vi "Orbit.vi"(11 "Input Velocities":T2) -> (3 "Output Velocities":T2)   [LabVIEW 2025]
uses:
  swerve-template/Type Definitions/Data/Robot Velocities.ctl
  <vilib>/Analysis/coordinate.llb/Angle Units.ctl
  <vilib>/Analysis/coordinate.llb/Angle Range (Degree).ctl
  <vilib>/Analysis/coordinate.llb/Wrap Angle (scalar).vi
  <vilib>/Rock Robotics/Network Tables/NT Read Integer.vi
  <vilib>/Rock Robotics/Network Tables/NT Read Float Array.vi
  <vilib>/addons/control/pid/pid.llb/PID Advanced (DBL).vi
  <vilib>/addons/control/pid/NI_PID_pid.lvlib
  <vilib>/Analysis/NI_AAL_Angle.lvlib
panel:
  in  "test values":sgl[](array[numeric])
  out "radial_vel":dbl format="%.2f"
  in  "Radius PID gains":T1={"proportional gain (Kc)"=0.01, "integral time (Ti, min)"=0.0, "derivative time (Td, min)"=0.0}
  out "radius_error":dbl
  out "desired_radius":dbl
  in  "k_radius":dbl=0.1
  out "driver_tangential_vel":dbl
  out "driver_radial_vel":dbl
  out "bearing_wrapped":dbl
  out "bearing_correction":dbl format="%.2f"
  in  "Heading PID gains":T1={"proportional gain (Kc)"=0.03, "integral time (Ti, min)"=0.0, "derivative time (Td, min)"=0.0}
  out "angular_vel_orbit":dbl
  out "desired_tangential_vel":dbl
  out "desired_radial_vel":dbl
  out "yaw":sgl
  out "curr_radius":sgl
  out "y":sgl
  out "x":sgl
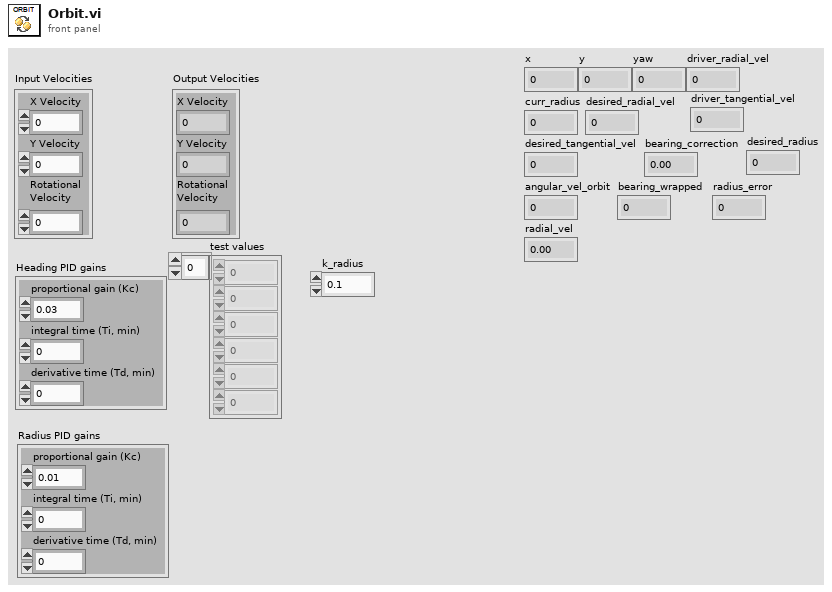
[diagram p1: front panel]
types:
  T1 = cluster{"proportional gain (Kc)":dbl, "integral time (Ti, min)":dbl, "derivative time (Td, min)":dbl}
  T2 = typedef "Robot Velocities.ctl" = cluster{"X Velocity":dbl, "Y Velocity":dbl, "Rotational \nVelocity":dbl}
  T3 = typedef "NI_AAL_Angle.lvlib/Angle Range (Degree).ctl" = u16
  T4 = typedef "NI_AAL_Angle.lvlib/Angle Units.ctl" = i32
  T5 = cluster{"X Velocity":dbl, "Y Velocity":dbl, "Rotational \nVelocity":dbl}
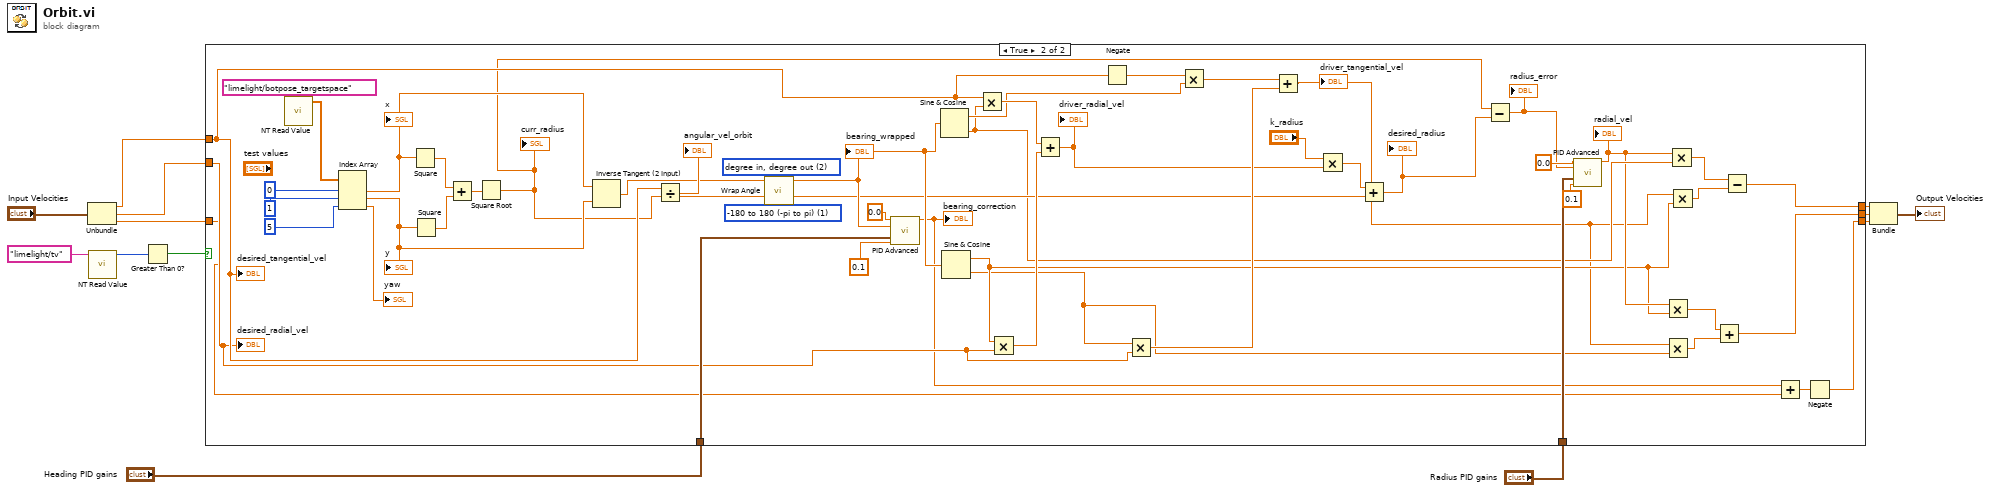
[diagram p0: block diagram]
diagram:
  n1 = Unbundle("Input Velocities") -> ("X Velocity"=w10:dbl, "Y Velocity"=w9:dbl, "Rotational \nVelocity"=w8:dbl)
  n2 = call-poly <vilib>:"NT Read Value.vi"("name"="limelight/tv") -> ("value"=w11:i64)  [unwired: 8 in, 2 out]
  n3 = Greater Than 0?(x=w11) -> (x > 0?=w1:bool)
  n4 = case shown="True" w1 {
    tunnel: w10 -> [w16 w48]
    tunnel: w9 -> [w15 w45]
    tunnel: w8 -> [w14 w22]
    tunnel: [w16 w31] -> w7
    tunnel: [w15 w24] -> w6
    tunnel: [w14 w20] -> w5
    tunnel: "Heading PID gains" -> [_ w57]
    tunnel: "Radius PID gains" -> [_ w35]
    frame False {
    }
    frame True {
      w52 = T3 1 items=["none", "-180 to 180 (-pi to pi)", "0 to 360 (0 to 2pi)"] ("angle range")
      w54 = T4 2 items=["radian in, radian out", "radian in, degree out", "degree in, degree out", "degree in, radian out"] ("angle units")
      n5 = call-poly <vilib>:"NT Read Value.vi"("name"="limelight/botpose_targetspace") -> ("value"=w17:sgl[])  [unwired: 8 in, 2 out]
      n6 = Index Array(array=w17, index #1=0 ("index"), index #2=1 ("index"), index #3=5 ("index")) -> (element #1=w61:sgl, element #2=w60:sgl, element #3=→"yaw":sgl)
      "x" <- w61
      "y" <- w60
      n7 = Square(x=w61) -> (x^2=w63:sgl)
      n8 = Square(x=w60) -> (x^2=w62:sgl)
      n9 = Add(x=w63, y=w62) -> (x+y=w64:sgl)
      n10 = Square Root(x=w64) -> (sqrt(x)=w38:sgl)
      "curr_radius" <- w38
      n11 = Inverse Tangent (2 Input)(1:w60, 2:w61) -> (0:w53:sgl)
      n12 = Divide(x=w48, y=w38) -> (x/y=→"angular_vel_orbit":dbl)
      n13 = call-poly <vilib>:"Wrap Angle.vi"("angle units"=w54, "angle range"=w52, "angle in"=w53) -> ("angle out"=w50:dbl)  [unwired: 7 in, 1 out]
      "bearing_wrapped" <- w50
      n14 = call-poly <vilib>:"PID Advanced.vi"("setpoint"=0.0, "process variable"=w50, "PID gains"=w57, "dt (s)"=0.1) -> ("output"=w23:dbl)  [unwired: 10 in, 1 out]
      "bearing_correction" <- w23
      n15 = Sine & Cosine(0:w50) -> (1:w47:dbl, 2:w34:dbl)
      n16 = Sine & Cosine(0:w50) -> (1:w29:dbl, 2:w26:dbl)
      n17 = Multiply(x=w48, y=w34) -> (x*y=w51:dbl)
      n18 = Multiply(x=w29, y=w45) -> (x*y=w49:dbl)
      n19 = Add(x=w51, y=w49) -> (x+y=w42:dbl)
      "driver_radial_vel" <- w42
      n20 = Negate(x=w48) -> (-x=w46:dbl)
      n21 = Multiply(x=w26, y=w45) -> (x*y=w43:dbl)
      n22 = Multiply(x=w46, y=w47) -> (x*y=w44:dbl)
      n23 = Add(x=w44, y=w43) -> (x+y=w27:dbl)
      "driver_tangential_vel" <- w27
      n24 = Multiply(x="k_radius", y=w42) -> (x*y=w40:dbl)
      n25 = Add(x=w40, y=w38) -> (x+y=w39:dbl)
      "desired_radius" <- w39
      n26 = Subtract(x=w38, y=w39) -> (x-y=w36:dbl)
      "radius_error" <- w36
      n27 = call-poly <vilib>:"PID Advanced.vi"("setpoint"=0.0, "process variable"=w36, "PID gains"=w35, "dt (s)"=0.1) -> ("output"=w30:dbl)  [unwired: 10 in, 1 out]
      "radial_vel" <- w30
      n28 = Multiply(x=w30, y=w29) -> (x*y=w28:dbl)
      n29 = Multiply(x=w27, y=w26) -> (x*y=w25:dbl)
      n30 = Multiply(x=w30, y=w34) -> (x*y=w33:dbl)
      n31 = Multiply(x=w27, y=w29) -> (x*y=w32:dbl)
      n32 = Add(x=w28, y=w25) -> (x+y=w24:dbl)
      n33 = Subtract(x=w33, y=w32) -> (x-y=w31:dbl)
      n34 = Add(x=w23, y=w22) -> (x+y=w21:dbl)
      n35 = Negate(x=w21) -> (-x=w20:dbl)
      "desired_radial_vel" <- w45
      "desired_tangential_vel" <- w48
    }
  }
  n36 = Bundle("X Velocity"=w7, "Y Velocity"=w6, "Rotational \nVelocity"=w5) -> (→"Output Velocities":T5)  [unwired: 1 in]
